vi "Main.vi"(10 "Message Queue Notifier":refnum<notifier>, 11 "Zero Timeout Message Handler in":refnum<class "Zero Timeout Message Handler.lvclass">) -> ()   [LabVIEW 2024, in "Zero Timeout Message Handler.lvlib" / "Zero Timeout Message Handler.lvclass"]
uses:
  Zero Timeout Message Handler.lvclass
  ~Message/~Message.lvclass
  Zero Timeout Message Handler.lvclass/Zero Timeout Message Handler.ctl
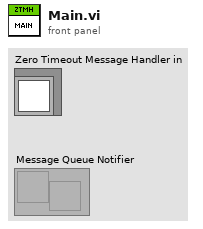
[diagram p1: front panel]
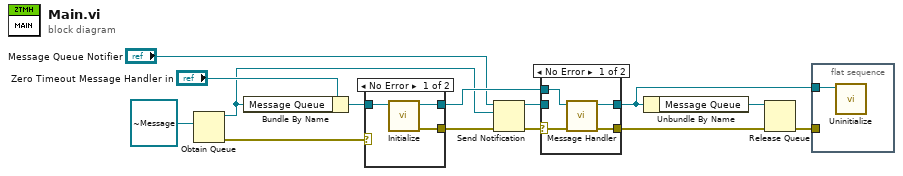
[diagram p0: block diagram]
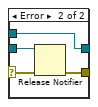
[diagram p2: hidden frame]
diagram:
  n1 = Obtain Queue(element data type=refnum<class "~Message.lvclass"> refnum ("Zero Timeout Message Handler.lvlib:~Message.lvclass")) -> (queue out=w1:refnum<queue>, error out=w6:errorcluster)  [unwired: 4 in, 1 out]
  n2 = Bundle By Name(cluster="Zero Timeout Message Handler in", "Message Queue"=w1) -> (w12:refnum<class "Zero Timeout Message Handler.lvclass">)
  n3 = case shown="No Error" w6 {
    selector: w6 -> [_ w19]
    tunnel: [w17 w19] -> w8
    tunnel: [w16 w18] -> w14
    tunnel: w12 -> [w15 w18]
    frame No Error {
      n4 = call-dynamic "Initialize.vi"("Zero Timeout Message Handler in"=w15) -> ("error out"=w17:errorcluster, "Zero Timeout Message Handler out"=w16:refnum<class "Zero Timeout Message Handler.lvclass">)  [unwired: 9 in]
    }
    frame Error {
    }
  }
  n5 = Send Notification(notification=w1, notifier="Message Queue Notifier", error in (no error)=w8) -> (notifier out=w9:refnum<notifier>, error out=w7:errorcluster)
  n6 = case shown="No Error" w7 {
    selector: w7 -> [w20 w27]
    tunnel: w14 -> [w23 w25]
    tunnel: [w22 w26] -> w4
    tunnel: [w21 w25] -> w3
    tunnel: w9 -> [_ w24]
    frame No Error {
      n7 = call "Message Handler.vi"("error in (no error)"=w20, "Zero Timeout Message Handler in"=w23) -> ("error out"=w22:errorcluster, "Zero Timeout Message Handler out"=w21:refnum<class "Zero Timeout Message Handler.lvclass">)  [unwired: 8 in]
    }
    frame Error {
      n8 = Release Notifier(notifier=w24, error in (no error)=w27) -> (error out=w26:errorcluster)  [unwired: 1 in, 2 out]
    }
  }
  n9 = Unbundle By Name(w3) -> ("Message Queue"=w5:refnum<queue>)
  n10 = Release Queue(queue=w5, error in (no error)=w4) -> (error out=w2:errorcluster)  [unwired: 1 in, 2 out]
  n11 = flat-sequence {
    tunnel: w3 -> [w28]
    tunnel: w2 -> [_]
    frame #0 {
      n12 = call-dynamic "Uninitialize.vi"("Zero Timeout Message Handler in"=w28) -> ()  [unwired: 10 in, 1 out]
    }
  }
